vi "IPS Parse Status.vi"(7 "X String":string="X42A1C2H5M12P21\r") -> (2 "X Strings":T1, 3 "X Cluster":T8={"System 1"=enum."Normal", "System 2"=enum."Outside Positive Current Limi", "Activity"=enum."Hold", "Switch Heater"=enum."No Switch Fitted", "Mode 1"=enum."Amps Fast", "Mode 2"=enum."At Rest"})   [LabVIEW 2016, in "IPS-120.lvlib"]
uses:
  IPS-120.lvlib
  Typedefs/Read X - Cluster.ctl
  Typedefs/Read System 1 - Enum.ctl
  Typedefs/Read System 2 - Enum.ctl
  Typedefs/Read Activity - Enum.ctl
  Typedefs/Read Switch Heater - Enum.ctl
  Typedefs/Read Mode 1 - Enum.ctl
  Typedefs/Read Mode 2 - Enum.ctl
panel:
  out "Mode 2":T2
  out "Mode 1":T3
  out "Switch Heater":T4
  out "Activity":T5
  out "System 2":T6
  out "System 1":T7
  out "System":string="42"
  out "Mode":string="12"
  out "Activity":i32=1
  out "Switch Heater":i32=5
  out "System":string="X42"
  out "Activity":string="A1"
  out "LOC/REM":string="C2"
  out "Switch Heater":string="H5"
  out "Mode":string="M12"
  out "Polarity":string="P21\r"
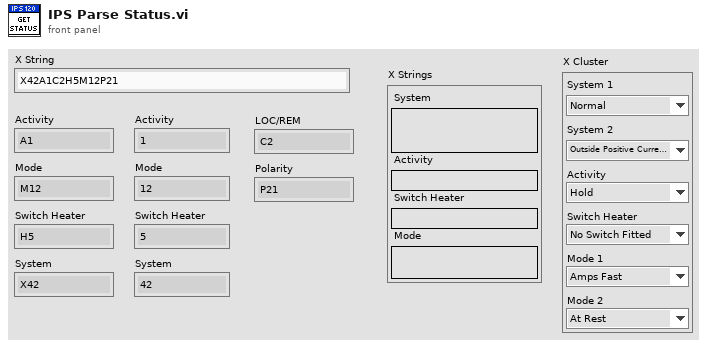
[diagram p1: front panel]
types:
  T1 = cluster{"System":string, "Activity":string, "Switch Heater":string, "Mode":string}
  T2 = typedef "IPS-120.lvlib/Read Mode 2 - Enum.ctl" = enum16{"At Rest", "Sweeping", "Sweep Limiting", "Sweeping & Sweep Limiting"}
  T3 = typedef "IPS-120.lvlib/Read Mode 1 - Enum.ctl" = enum16{"Amps Fast", "Tesla Fast", "Amps Slow", "Tesla Slow"}
  T4 = typedef "IPS-120.lvlib/Read Switch Heater - Enum.ctl" = enum16{"Off Magnet at Zero", "On", "Off Magnet at Field", "Heater Fault", "No Switch Fitted"}
  T5 = typedef "IPS-120.lvlib/Read Activity - Enum.ctl" = enum16{"Hold", "To Set Point", "To Zero", "Clamped"}
  T6 = typedef "IPS-120.lvlib/Read System 2 - Enum.ctl" = enum16{"Normal", "On Positive Voltage Limit", "On Negative Voltage Limit", "Outside Negative Current Limit", "Outside Positive Current Limi"}
  T7 = typedef "IPS-120.lvlib/Read System 1 - Enum.ctl" = enum16{"Normal", "Quenched", "Over Heated", "Warming Up", "Fault"}
  T8 = typedef "IPS-120.lvlib/Read X - Cluster.ctl" = cluster{"System 1":T7, "System 2":T6, "Activity":T5, "Switch Heater":T4, "Mode 1":T3, "Mode 2":T2}
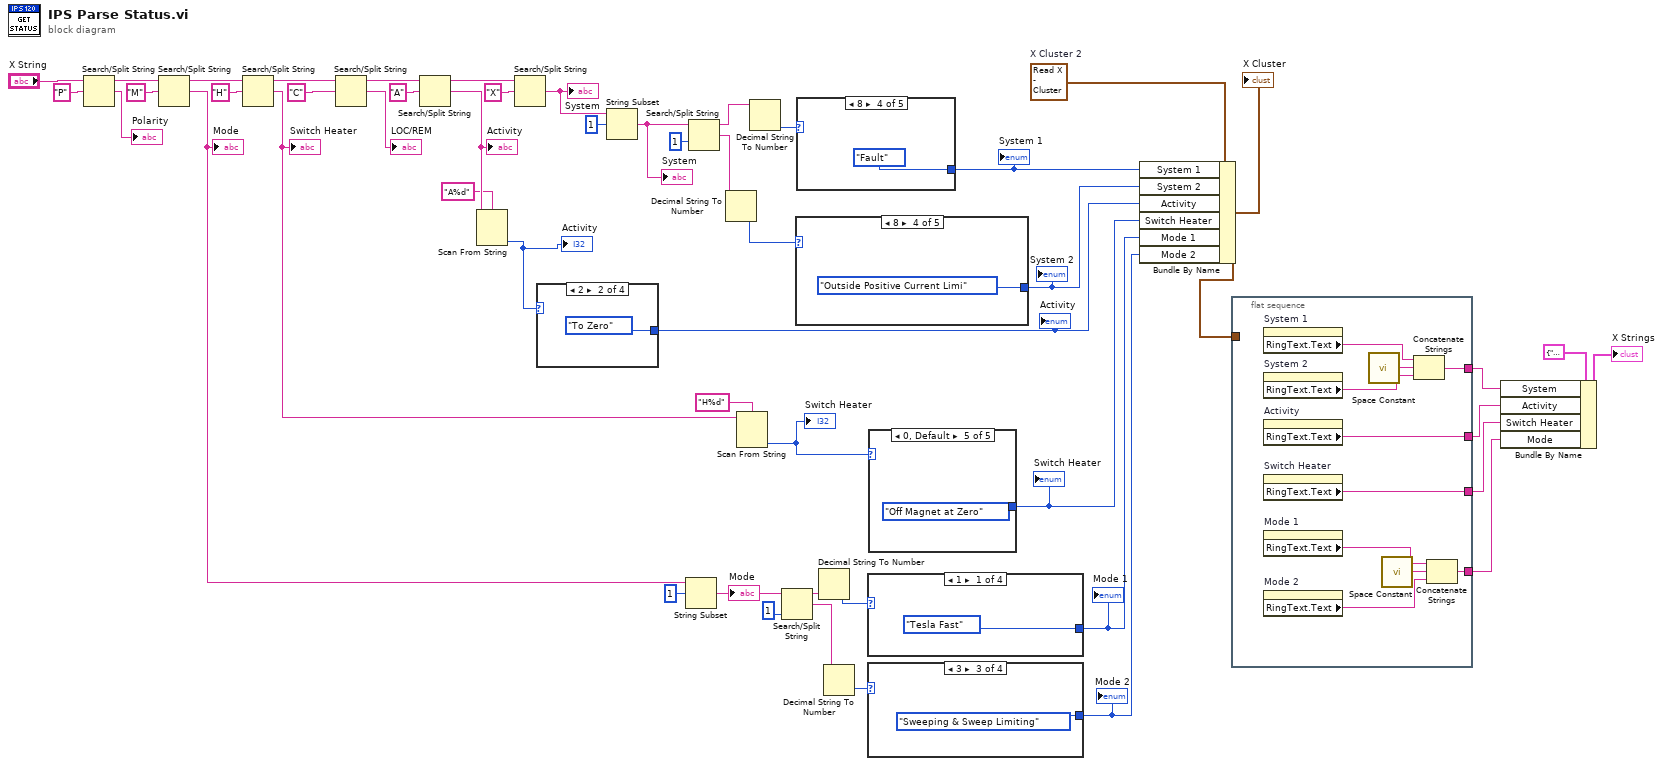
[diagram p0: block diagram]
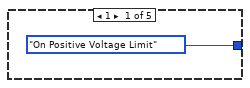
[diagram p2: hidden frame]
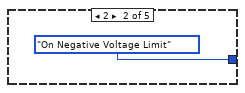
[diagram p3: hidden frame]
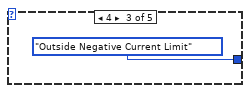
[diagram p4: hidden frame]
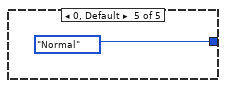
[diagram p5: hidden frame]
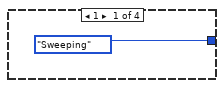
[diagram p6: hidden frame]
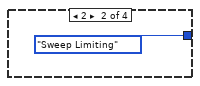
[diagram p7: hidden frame]
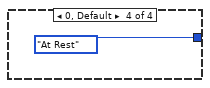
[diagram p8: hidden frame]
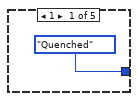
[diagram p9: hidden frame]
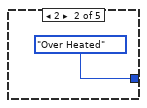
[diagram p10: hidden frame]
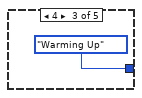
[diagram p11: hidden frame]
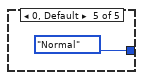
[diagram p12: hidden frame]
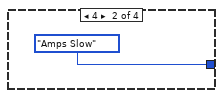
[diagram p13: hidden frame]
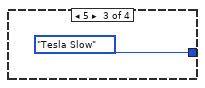
[diagram p14: hidden frame]
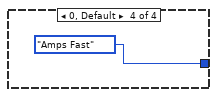
[diagram p15: hidden frame]
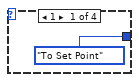
[diagram p16: hidden frame]
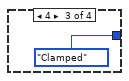
[diagram p17: hidden frame]
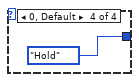
[diagram p18: hidden frame]
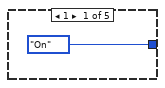
[diagram p19: hidden frame]
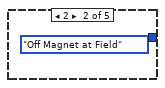
[diagram p20: hidden frame]
diagram:
  w14 = T8 {"System 1"=enum."Normal", "System 2"=enum."Outside Positive Current Limi", "Activity"=enum."Hold", "Switch Heater"=enum."No Switch Fitted", "Mode 1"=enum."Amps Fast", "Mode 2"=enum."At Rest"}  # X Cluster 2
  n1 = Search/Split String(string="X String", search string/char (-)="P") -> (substring before match=w47:string, match + rest of string=→"Polarity":string)  [unwired: 1 in, 1 out]
  n2 = Search/Split String(string=w47, search string/char (-)="M") -> (substring before match=w46:string, match + rest of string=w32:string)  [unwired: 1 in, 1 out]
  "Mode" <- w32
  n3 = Search/Split String(string=w46, search string/char (-)="H") -> (substring before match=w44:string, match + rest of string=w36:string)  [unwired: 1 in, 1 out]
  "Switch Heater" <- w36
  n4 = Search/Split String(string=w44, search string/char (-)="C") -> (substring before match=w42:string, match + rest of string=→"LOC/REM":string)  [unwired: 1 in, 1 out]
  n5 = Search/Split String(string=w42, search string/char (-)="A") -> (substring before match=w39:string, match + rest of string=w34:string)  [unwired: 1 in, 1 out]
  "Activity" <- w34
  n6 = Scan From String(format string="A%d", input string=w34) -> (output 1=w15:i32)  [unwired: 3 in, 3 out]
  "Activity" <- w15
  n7 = Search/Split String(string=w39, search string/char (-)="X") -> (match + rest of string=w29:string)  [unwired: 1 in, 2 out]
  "System" <- w29
  n8 = case shown="2" w15 {
    tunnel: [Read_Activity_-_Enum."To Set Point" ("Activity") Read_Activity_-_Enum."To Zero" ("Activity") Read_Activity_-_Enum."Clamped" ("Activity") Read_Activity_-_Enum."Hold" ("Activity")] -> w11
    frame 1 {
    }
    frame 2 {
    }
    frame 4 {
    }
    frame 0, Default {
    }
  }
  "Activity" <- w11
  n9 = String Subset(string=w29, offset (0)=1) -> (substring=w25:string)  [unwired: 1 in]
  "System" <- w25
  n10 = String Subset(string=w32, offset (0)=1) -> (substring=w16:string)  [unwired: 1 in]
  "Mode" <- w16
  n11 = Search/Split String(string=w25, offset (0)=1) -> (substring before match=w20:string, match + rest of string=w22:string)  [unwired: 1 in, 1 out]
  n12 = Decimal String To Number(string=w22) -> (number=w21:i32)  [unwired: 2 in, 1 out]
  n13 = Scan From String(format string="H%d", input string=w36) -> (output 1=w24:i32)  [unwired: 3 in, 3 out]
  "Switch Heater" <- w24
  n14 = Decimal String To Number(string=w20) -> (number=w23:i32)  [unwired: 2 in, 1 out]
  n15 = Search/Split String(string=w16, offset (0)=1) -> (substring before match=w28:string, match + rest of string=w27:string)  [unwired: 1 in, 1 out]
  n16 = case shown="8" w21 {
    tunnel: [Read_System_2_-_Enum."On Positive Voltage Limit" ("System 2") Read_System_2_-_Enum."On Negative Voltage Limit" ("System 2") Read_System_2_-_Enum."Outside Negative Current Limit" ("System 2") Read_System_2_-_Enum."Outside Positive Current Limi" ("System 2") Read_System_2_-_Enum."Normal" ("System 2")] -> w12
    frame 1 {
    }
    frame 2 {
    }
    frame 4 {
    }
    frame 8 {
    }
    frame 0, Default {
    }
  }
  "System 2" <- w12
  n17 = case shown="8" w23 {
    tunnel: [Read_System_1_-_Enum."Quenched" ("System 1") Read_System_1_-_Enum."Over Heated" ("System 1") Read_System_1_-_Enum."Warming Up" ("System 1") Read_System_1_-_Enum."Fault" ("System 1") Read_System_1_-_Enum."Normal" ("System 1")] -> w13
    frame 1 {
    }
    frame 2 {
    }
    frame 4 {
    }
    frame 8 {
    }
    frame 0, Default {
    }
  }
  "System 1" <- w13
  n18 = Decimal String To Number(string=w28) -> (number=w19:i32)  [unwired: 2 in, 1 out]
  n19 = Decimal String To Number(string=w27) -> (number=w18:i32)  [unwired: 2 in, 1 out]
  n20 = case shown="1" w19 {
    tunnel: [Read_Mode_1_-_Enum."Tesla Fast" ("Mode 1") Read_Mode_1_-_Enum."Amps Slow" ("Mode 1") Read_Mode_1_-_Enum."Tesla Slow" ("Mode 1") Read_Mode_1_-_Enum."Amps Fast" ("Mode 1")] -> w9
    frame 1 {
    }
    frame 4 {
    }
    frame 5 {
    }
    frame 0, Default {
    }
  }
  "Mode 1" <- w9
  n21 = case shown="3" w18 {
    tunnel: [Read_Mode_2_-_Enum."Sweeping" ("Mode 2") Read_Mode_2_-_Enum."Sweep Limiting" ("Mode 2") Read_Mode_2_-_Enum."Sweeping & Sweep Limiting" ("Mode 2") Read_Mode_2_-_Enum."At Rest" ("Mode 2")] -> w8
    frame 1 {
    }
    frame 2 {
    }
    frame 3 {
    }
    frame 0, Default {
    }
  }
  "Mode 2" <- w8
  n22 = case shown="0, Default" w24 {
    tunnel: [Read_Switch_Heater_-_Enum."On" ("Read Switch Heater") Read_Switch_Heater_-_Enum."Off Magnet at Field" ("Read Switch Heater") Read_Switch_Heater_-_Enum."Heater Fault" ("Read Switch Heater") Read_Switch_Heater_-_Enum."No Switch Fitted" ("Read Switch Heater") Read_Switch_Heater_-_Enum."Off Magnet at Zero" ("Read Switch Heater")] -> w10
    frame 1 {
    }
    frame 2 {
    }
    frame 5 {
    }
    frame 8 {
    }
    frame 0, Default {
    }
  }
  "Switch Heater" <- w10
  n23 = Bundle By Name(cluster=w14, "System 1"=w13, "System 2"=w12, "Activity"=w11, "Switch Heater"=w10, "Mode 1"=w9, "Mode 2"=w8) -> (w7:T8)
  "X Cluster" <- w7
  n24 = flat-sequence {
    tunnel: w7 -> [_]
    tunnel: [w81] -> w5
    tunnel: [w80] -> w2
    tunnel: [w79] -> w3
    tunnel: [w78] -> w4
    frame #0 {
      n25 = property on="System 1" class="Enum (strict)"() -> ("RingText.Text"=w86:string)  [unwired: 2 in, 2 out]
      n26 = property on="System 2" class="Enum (strict)"() -> ("RingText.Text"=w85:string)  [unwired: 2 in, 2 out]
      n27 = property on="Activity" class="Enum (strict)"() -> ("RingText.Text"=w80:string)  [unwired: 2 in, 2 out]
      n28 = property on="Switch Heater" class="Enum (strict)"() -> ("RingText.Text"=w79:string)  [unwired: 2 in, 2 out]
      n29 = property on="Mode 1" class="Enum (strict)"() -> ("RingText.Text"=w83:string)  [unwired: 2 in, 2 out]
      n30 = property on="Mode 2" class="Enum (strict)"() -> ("RingText.Text"=w82:string)  [unwired: 2 in, 2 out]
      n31 = call <vilib>:"Space Constant.vi"() -> ("String"=w87:string)
      n32 = call <vilib>:"Space Constant.vi"() -> ("String"=w84:string)
      n33 = Concatenate Strings(w86, w87, w85) -> (w81:string)
      n34 = Concatenate Strings(w83, w84, w82) -> (w78:string)
    }
  }
  n35 = Bundle By Name(cluster=T1 {"System"="", "Activity"="", "Switch Heater"="", "Mode"=""} ("X Strings 2"), "System"=w5, "Activity"=w2, "Switch Heater"=w3, "Mode"=w4) -> (→"X Strings":T1)
